vi "Stop.vi"(8 "error in":errorcluster, 11 "NEOXID480HTA in":refnum<class "NEOXID480.lvclass">) -> (0 "error out":errorcluster, 3 "NEOXID480HTA out":refnum<class "NEOXID480.lvclass">)   [LabVIEW 2024, in "NEOXID480.lvclass"]
uses:
  NEOXID480.lvclass
  NEOXID480.lvclass/NEOXID480.ctl
  Source/Interfaces/IRunnable/IRunnable.lvclass
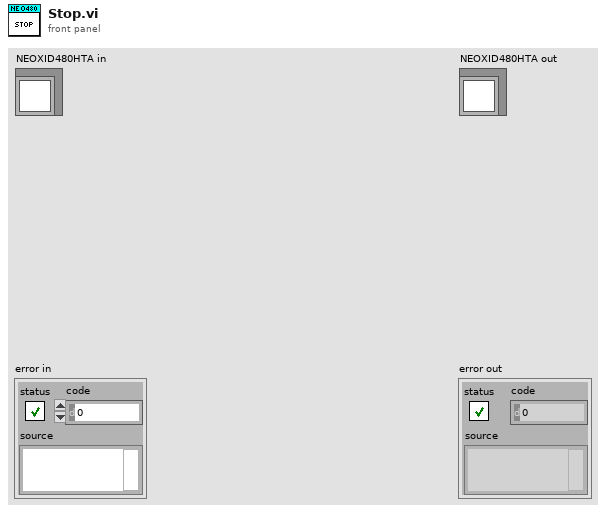
[diagram p1: front panel]
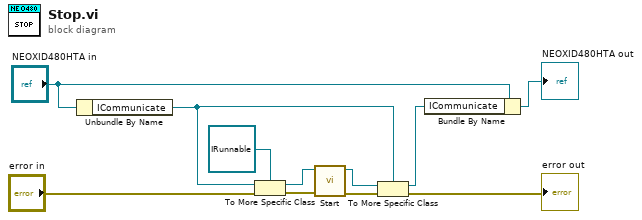
[diagram p0: block diagram]
diagram:
  n1 = Unbundle By Name("NEOXID480HTA in") -> ("ICommunicate"=w6:refnum<class "ICommunicate.lvclass">)
  n2 = To More Specific Class(target class=refnum<class "IRunnable.lvclass"> refnum ("IRunnable.lvclass"), reference=w6, error in="error in") -> (specific class reference=w10:refnum<class "IRunnable.lvclass">, error out=w9:errorcluster)
  n3 = call-dynamic "Start.vi"("error in"=w9, "IRunnable in"=w10) -> ("error out"=w8:errorcluster, "IRunnable out"=w7:refnum<class "IRunnable.lvclass">)  [unwired: 8 in]
  n4 = To More Specific Class(target class=w6, reference=w7, error in=w8) -> (specific class reference=w5:refnum<class "ICommunicate.lvclass">, error out=→"error out":errorcluster)
  n5 = Bundle By Name(cluster="NEOXID480HTA in", "ICommunicate"=w5) -> (→"NEOXID480HTA out":refnum<class "NEOXID480.lvclass">)
